vi "REPORT_OPRTN_set_filter_values.vi"(4 "REPORT_all_info":T1, 6 "gears":string[][](array[string]), 11 "error_in":errorcluster) -> (3 "error_out":errorcluster)   [LabVIEW 2019]
uses:
  FGV/REPORTS_records_display/REPORTS_all_info.ctl
  GEAR/typedef/REPORT_GEAR_all_info.ctl
  GEAR/typedef/REPORT_GEAR_header_data_display.ctl
  GEAR/typedef/REPORT_GEAR_statuses.ctl
  DATES/typedef/REPORT_DATES_all_info.ctl
  DATES/typedef/REPORT_DATES_statuses.ctl
  PRODUCTION_BATCH/typedef/REPORT_PBATCH_all_info.ctl
  typedef/REPORT_OPRTN_all_info.ctl
  CONFIG_HISTORY/typedef/REPORT_CFG_all_info.ctl
  CONFIG_HISTORY/typedef/REPORT_CFG_types.ctl
  AUDIT/typedef/REPORT_AUDIT_all_info.ctl
  OK_NOK_COUNT/typedef/REPORT_OKNOK_all_info.ctl
  REWORKS/typedef/REPORT_REWORKS_all_info.ctl
  PACE/typedef/REPORT_PACE_all_info.ctl
  CUSTOMER_BATCH/typedef/REPORT_CBATCH_all_info.ctl
  GEAR_COMPONENTS/typedef/REPORT_CMPNT_all_info.ctl
  FGV/REPORTS_records_display/REPORTS_references.ctl
  <userlib>/_OpenG.lib/array/array.llb/Remove Duplicates from 1D Array (String)__ogtk.vi
panel:
  # "GEAR INFO SUMMARY"
  # "GEAR INFO SUMMARY"
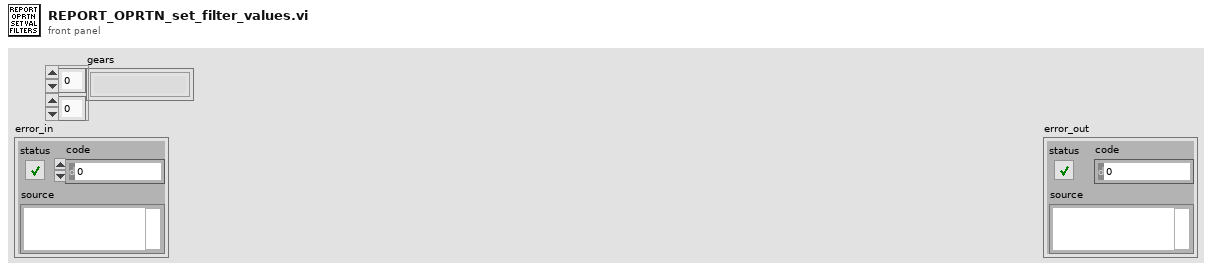
[diagram p1: front panel]
types:
  T1 = typedef "REPORTS_all_info.ctl" = cluster{"REPORT_GEAR_all_info":T2, "REPORT_DATES_all_info":T5, "REPORT_PBATCH_all_info":T7, "REPORT_OPRTN_all_info":T8, "REPORT_CFG_all_info":T9, "REPORT_AUDIT_all_info":T11, "REPORT_OKNOK_all_info":T12, "REPORT_REWORKS_all_info":T13, "REPORT_PACE_all_info":T14, "REPORT_CBATCH_all_info":T15, "REPORT_CMPNT_all_info":T16, "REPORTS_references":T17}
  T2 = typedef "REPORT_GEAR_all_info.ctl" = cluster{"serial":string, "filter_OP":string, "REPORT_GEAR_header":T3, "operations":string[][], "operation_statuses":T4[], "results":string[][], "result_statuses":T4[], "batches":string[][], "batch_statuses":T4[], "column_headers":string[], "displayed_rows":string[][], "displayed_statuses":T4[], "column_widths":i16[]}
  T3 = typedef "REPORT_GEAR_header_data_display.ctl" = cluster{"ID":string, "creation_time":string, "last_station":string, "last_status":string, "pinion_serial":string, "batch_code":string}
  T4 = typedef "REPORT_GEAR_statuses.ctl" = enum16{"OP_OK_hide", "OP_OK_show", "OP_NOK_hide", "OP_NOK_show", "OP_interrupted_hide", "OP_interrupted_show", "OP_in_operation_hide", "OP_in_operation_show", "OP_unexpected_hide", "OP_unexpected_show", "RE_REAL_OK", "RE_REAL_NOK", "RE_STRING", "RE_sub_header", "RE_no_data", "RE_unexpected", "BA_sub_header", "BA_data", "BA_no_data"}
  T5 = typedef "REPORT_DATES_all_info.ctl" = cluster{"date_start":string, "date_end":string, "time_start":string, "time_end":string, "filter_last_OP":string, "filter_last_status":string, "gears":string[][], "gears_statuses":T6[], "column_headers":string[], "displayed_rows":string[][], "displayed_statuses":T6[], "column_widths":i16[], "active_page":i32}
  T6 = typedef "REPORT_DATES_statuses.ctl" = enum16{"GEAR_OK", "GEAR_NOK", "GEAR_interrupted", "GEAR_in_operation", "GEAR_unexpected"}
  T7 = typedef "REPORT_PBATCH_all_info.ctl" = cluster{"batch_no":string, "filter_last_OP":string, "filter_last_status":string, "gears":string[][], "gears_statuses":T6[], "column_headers":string[], "displayed_rows":string[][], "displayed_statuses":T6[], "column_widths":i16[], "active_page":i32}
  T8 = typedef "REPORT_OPRTN_all_info.ctl" = cluster{"OP":string, "date_start":string, "date_end":string, "time_start":string, "time_end":string, "filter_last_status":string, "no_of_static_columns":i32, "operations":string[][], "operations_statuses":T6[], "column_headers":string[], "archivisation_description":string[][], "displayed_rows":string[][], "displayed_statuses":T6[], "column_widths":i16[], "hidden_columns":i32[], "active_page":i32}
  T9 = typedef "REPORT_CFG_all_info.ctl" = cluster{"type":T10, "date_start":string, "date_end":string, "time_start":string, "time_end":string, "filter_OP":string, "records":string[][], "column_headers":string[], "displayed_rows":string[][], "column_widths":i16[], "active_page":i32}
  T10 = typedef "REPORT_CFG_types.ctl" = enum16{"REFERENCE", "ARCHIVISATION", "USERS"}
  T11 = typedef "REPORT_AUDIT_all_info.ctl" = cluster{"date_start":string, "date_end":string, "time_start":string, "time_end":string, "filter_OP":string, "filter_status":string, "records":string[][], "record_statuses":T6[], "column_headers":string[], "displayed_rows":string[][], "displayed_statuses":T6[], "column_widths":i16[], "active_page":i32}
  T12 = typedef "REPORT_OKNOK_all_info.ctl" = cluster{"date_start":string, "date_end":string, "time_start":string, "time_end":string, "records":string[][], "column_headers":string[], "column_widths":i16[]}
  T13 = typedef "REPORT_REWORKS_all_info.ctl" = cluster{"date_start":string, "date_end":string, "time_start":string, "time_end":string, "from_OP":string, "to_OP":string, "records":string[][], "record_statuses":T6[], "column_headers":string[], "displayed_rows":string[][], "displayed_statuses":T6[], "column_widths":i16[], "active_page":i32}
  T14 = typedef "REPORT_PACE_all_info.ctl" = cluster{"date_start":string, "date_end":string, "time_start":string, "time_end":string, "low_limit":u16, "high_limit":u16, "records":string[][], "column_headers":string[], "column_widths":i16[]}
  T15 = typedef "REPORT_CBATCH_all_info.ctl" = cluster{"batch_code":string, "records":string[][], "record_statuses":T6[], "column_headers":string[], "displayed_rows":string[][], "displayed_statuses":T6[], "column_widths":i16[], "active_page":i32}
  T16 = typedef "REPORT_CMPNT_all_info.ctl" = cluster{"gear_serial":string, "records":string[][], "column_headers":string[], "displayed_rows":string[][], "column_widths":i16[], "active_page":i32}
  T17 = typedef "REPORTS_references.ctl" = cluster{"front_panel_reference":refnum<vi>, "SQL_listbox_reference":refnum<vi>, "REPORT_page_first":refnum<vi>, "REPORT_page_previous":refnum<vi>, "REPORT_page_next":refnum<vi>, "REPORT_page_last":refnum<vi>, "REPORT_page_counter":refnum<vi>, "REPORT_GEAR_serial":refnum<vi>, "REPORT_GEAR_serial_display":refnum<vi>, "REPORT_GEAR_station":refnum<vi>, "REPORT_GEAR_header_data_display":refnum<vi>, "REPORT_DATES_start":refnum<vi>, "REPORT_DATES_end":refnum<vi>, "REPORT_DATES_time_start":refnum<vi>, "REPORT_DATES_time_end":refnum<vi>, "REPORT_DATES_order_selection":refnum<vi>, "REPORT_DATES_last_OP":refnum<vi>, "REPORT_DATES_last_status":refnum<vi>, "REPORT_PBATCH_batch_no":refnum<vi>, "REPORT_PBATCH_order_selection":refnum<vi>, "REPORT_PBATCH_last_op":refnum<vi>, "REPORT_PBATCH_last_status":refnum<vi>, "REPORT_OPRTN_operation":refnum<vi>, "REPORT_OPRTN_start":refnum<vi>, "REPORT_OPRTN_end":refnum<vi>, "REPORT_OPRTN_time_start":refnum<vi>, "REPORT_OPRTN_time_end":refnum<vi>, "REPORT_OPRTN_order_selection":refnum<vi>, "REPORT_OPRTN_last_status":refnum<vi>, "REPORT_CFG_type":refnum<vi>, "REPORT_CFG_start":refnum<vi>, "REPORT_CFG_end":refnum<vi>, "REPORT_CFG_time_start":refnum<vi>, "REPORT_CFG_time_end":refnum<vi>, "REPORT_CFG_order_selection":refnum<vi>, "REPORT_CFG_op_filter":refnum<vi>, "REPORT_AUDIT_start":refnum<vi>, "REPORT_AUDIT_end":refnum<vi>, "REPORT_AUDIT_time_start":refnum<vi>, "REPORT_AUDIT_time_end":refnum<vi>, "REPORT_AUDIT_order_selection":refnum<vi>, "REPORT_AUDIT_op_filter":refnum<vi>, "REPORT_AUDIT_status_filter":refnum<vi>, "REPORT_OKNOK_start":refnum<vi>, "REPORT_OKNOK_end":refnum<vi>, "REPORT_OKNOK_time_start":refnum<vi>, "REPORT_OKNOK_time_end":refnum<vi>, "REPORT_REWORKS_start":refnum<vi>, "REPORT_REWORKS_end":refnum<vi>, "REPORT_REWORKS_time_start":refnum<vi>, "REPORT_REWORKS_time_end":refnum<vi>, "REPORT_REWORKS_from_OP":refnum<vi>, "REPORT_REWORKS_to_OP":refnum<vi>, "REPORT_REWORKS_order_selection":refnum<vi>, "REPORT_PACE_start":refnum<vi>, "REPORT_PACE_end":refnum<vi>, "REPORT_PACE_time_start":refnum<vi>, "REPORT_PACE_time_end":refnum<vi>, "REPORT_PACE_low_limit":refnum<vi>, "REPORT_PACE_high_limit":refnum<vi>, "REPORT_CBATCH_batch_code":refnum<vi>, "REPORT_CBATCH_order_selection":refnum<vi>, "REPORT_CMPNT_gear_serial":refnum<vi>}
  T18 = enum8{"Enabled", "Disabled", "Disabled and Grayed Out"}
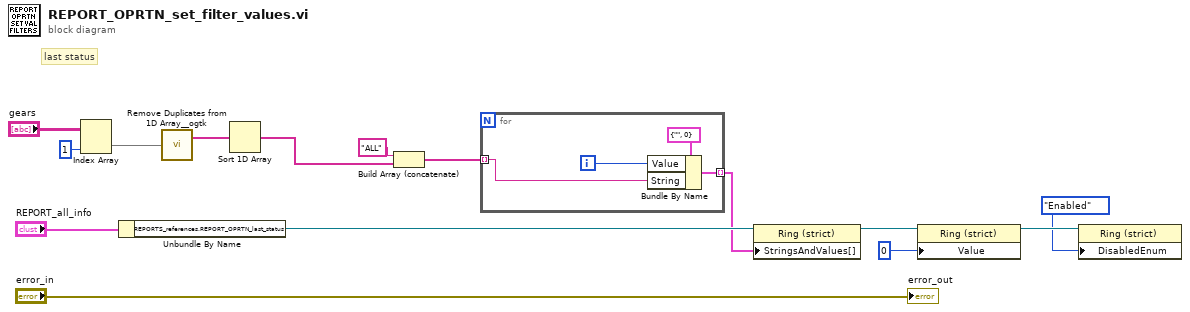
[diagram p0: block diagram]
diagram:
  # "last status"
  n1 = Index Array(array="gears", index (col)=1) -> (element=w11:string[])  [unwired: 1 in]
  n2 = Unbundle By Name("REPORT_all_info") -> ("REPORTS_references.REPORT_OPRTN_last_status"=w10:refnum<vi>)
  n3 = call-poly <userlib>:"Remove Duplicates from 1D Array__ogtk.vi"("Input Array"=w11) -> ("Output Array"=w8:string[])  [unwired: 1 out]
  n4 = Sort 1D Array(array=w8) -> (sorted array=w6:string[])
  n5 = Build Array (concatenate)("ALL" ("String"), w6) -> (w5:string[])
  n6 = for {
    tunnel: w5 -> [w16] mode=indexing
    tunnel: [w18] -> w9 mode=indexing
    i -> [w17]
    n7 = Bundle By Name(cluster=cluster{"String":string, "Value":u16} {"String"="", "Value"=0}, "Value"=w17, "String"=w16) -> (w18:cluster{"String":string, "Value":u16})
  }
  n8 = property class="Ring (strict)"(reference=w10, "StringsAndValues[]"=w9) -> (reference out=w4:refnum<vi>)  [unwired: 1 in, 1 out]
  n9 = property class="Ring (strict)"(reference=w4, "Value"=u16 0) -> (reference out=w3:refnum<vi>)  [unwired: 1 in, 1 out]
  n10 = property class="Ring (strict)"(reference=w3, "DisabledEnum"=T18."Enabled" ("Disabled")) -> ()  [unwired: 1 in, 2 out]
  "error_out" <- "error_in"
